vi "NI 9425 TASK.vi"(8 "error in":errorcluster, 11 "MODULE NAME":string="cDAQ_NICOTRAMod1") -> (0 "error out":errorcluster, 3 "task out":refnum<k21>)   [LabVIEW 2016]
uses:
  <vilib>/DAQmx/create/channels.llb/DAQmx Create Channel (DI-Digital Input).vi
  <resource>/objmgr/daqmx.rc
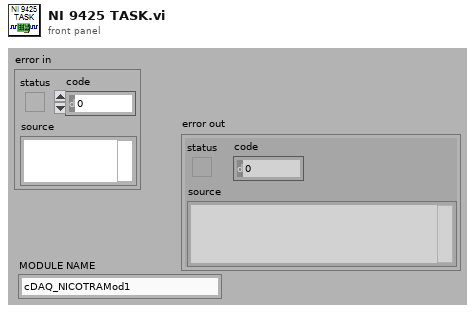
[diagram p1: front panel]
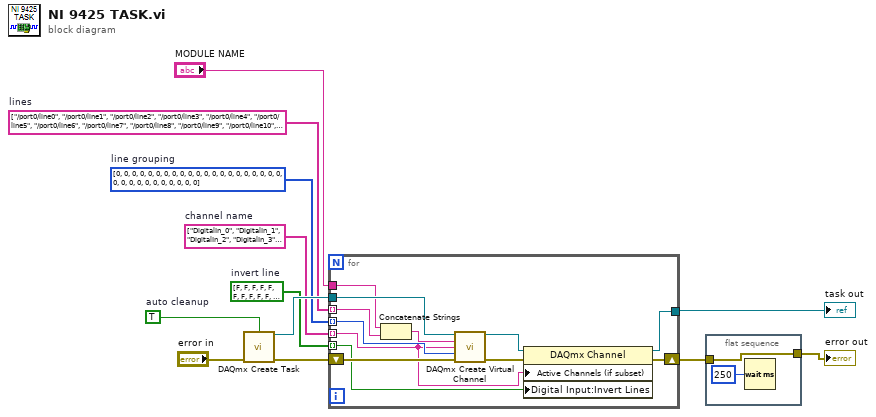
[diagram p0: block diagram]
diagram:
  w8 = bool[] [FALSE, FALSE, FALSE, FALSE, FALSE, FALSE, FALSE, FALSE, FALSE, FALSE, FALSE, FALSE, FALSE, FALSE, FALSE, FALSE, FALSE, FALSE, FALSE, FALSE, FALSE, FALSE, FALSE, FALSE, FALSE, FALSE, FALSE, FALSE, FALSE, FALSE, FALSE, FALSE]  # invert line
  w7 = i32[] [0, 0, 0, 0, 0, 0, 0, 0, 0, 0, 0, 0, 0, 0, 0, 0, 0, 0, 0, 0, 0, 0, 0, 0, 0, 0, 0, 0, 0, 0, 0, 0] items=["one channel for each line", "one channel for all lines"]  # line grouping
  w6 = string[] ["DigitalIn_0", "DigitalIn_1", "DigitalIn_2", "DigitalIn_3", "DigitalIn_4", "DigitalIn_5", "DigitalIn_6", "DigitalIn_7", "DigitalIn_8", "DigitalIn_9", "DigitalIn_10", "DigitalIn_11", "DigitalIn_12", "DigitalIn_13", "DigitalIn_14", "DigitalIn_15", "DigitalIn_16", "DigitalIn_17", "DigitalIn_18", "DigitalIn_19", "DigitalIn_20", "DigitalIn_21", "DigitalIn_22", "DigitalIn_23", "DigitalIn_24", "DigitalIn_25", "DigitalIn_26", "DigitalIn_27", "DigitalIn_28", "DigitalIn_29", "DigitalIn_30", "DigitalIn_31"]  # channel name
  w5 = string[] ["/port0/line0", "/port0/line1", "/port0/line2", "/port0/line3", "/port0/line4", "/port0/line5", "/port0/line6", "/port0/line7", "/port0/line8", "/port0/line9", "/port0/line10", "/port0/line11", "/port0/line12", "/port0/line13", "/port0/line14", "/port0/line15", "/port0/line16", "/port0/line17", "/port0/line18", "/port0/line19", "/port0/line20", "/port0/line21", "/port0/line22", "/port0/line23", "/port0/line24", "/port0/line25", "/port0/line26", "/port0/line27", "/port0/line28", "/port0/line29", "/port0/line30", "/port0/line31"]  # lines
  w10 = TRUE  # auto cleanup
  n1 = call <vilib>:"DAQmx Create Task.vi"("auto cleanup"=w10, "error in"="error in") -> ("task out"=w9:refnum<k21>, "error out"=w11:errorcluster)  [unwired: 12 in]
  n2 = for {
    tunnel: w9 -> [w24]
    tunnel: w8 -> [w19] mode=indexing
    tunnel: w7 -> [w22] mode=indexing
    tunnel: w6 -> [w18] mode=indexing
    tunnel: w5 -> [w15] mode=indexing
    tunnel: [w20] -> w4
    shift-right: [w16] -> w1
    shift-left: w11 -> [w23]
    tunnel: "MODULE NAME" -> [w14]
    n3 = Concatenate Strings(w14, w15) -> (w13:string)
    n4 = call-poly <vilib>:"DAQmx Create Virtual Channel.vi"("task in"=w24, "lines"=w13, "name to assign"=w18, "line grouping"=w22, "error in"=w23) -> ("task out"=w21:refnum<k21>, "error out"=w17:errorcluster)  [unwired: 9 in]
    n5 = property class="DAQmx Channel"(reference=w21, error in=w17, "Active Channels (if subset)"=w18, "Digital Input:Invert Lines"=w19) -> (reference out=w20:refnum<k21>, error out=w16:errorcluster)
  }
  "task out" <- w4
  n6 = flat-sequence {
    tunnel: [w25] -> w2
    tunnel: w1 -> [w25]
    frame #0 {
      n7 = Wait (ms)(milliseconds to wait=u32 250) -> ()  [unwired: 1 out]
    }
  }
  "error out" <- w2
